vi "Player Info.vi"(8 "Victory Speech":string="All your base are belong to us!!", 9 "Name":string, 11 "Coward in":refnum<class "Coward.lvclass">) -> (3 "Coward out":refnum<class "Coward.lvclass">)   [LabVIEW 2015, in "Coward.lvclass"]
uses:
  Coward.lvclass
  Formics/Formics.lvclass
panel:
  # "Set default values for these two string controls"
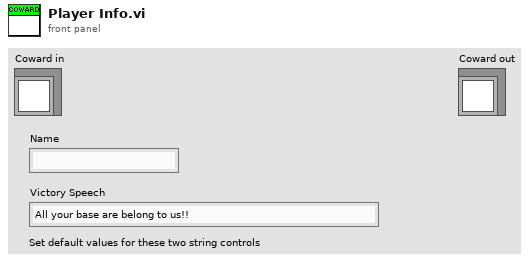
[diagram p1: front panel]
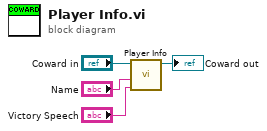
[diagram p0: block diagram]
diagram:
  n1 = call-parent "Player Info.vi"("Victory Speech"="Victory Speech", "Name"="Name", "Formics in"="Coward in") -> ("Formics out"=→"Coward out":refnum<class "Coward.lvclass">)  [unwired: 8 in]
